vi "Single Step Mode Status.vi"(0 "VISA resource name":refnum<visa-resource-name>, 11 "error in (no error)":errorcluster) -> (4 "VISA resource name out":refnum<visa-resource-name>, 6 "Single Step Mode Status":bool, 15 "error out":errorcluster)   [LabVIEW 2014, in "eec 6700.lvlib"]
doc: "Gets the single step mode status of the power source instrument.\n\nNote : supported in Program mode only."
uses:
  <instrlib>/eec 6700/eec 6700.lvlib
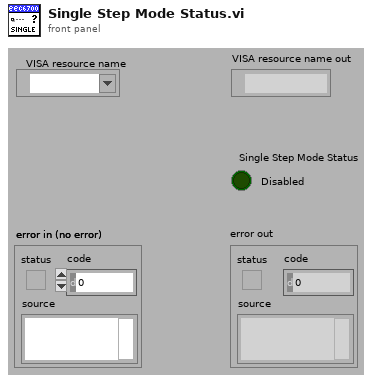
[diagram p1: front panel]
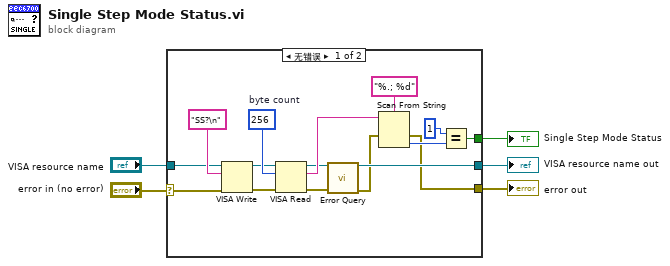
[diagram p0: block diagram]
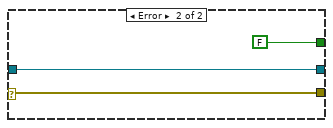
[diagram p2: hidden frame]
diagram:
  n1 = case shown="无错误" "error in (no error)" {
    selector: "error in (no error)" -> [w13 w23]
    tunnel: [w18 FALSE] -> w5
    tunnel: "VISA resource name" -> [w12 w24]
    tunnel: [w6 w23] -> w2
    tunnel: [w10 w24] -> w1
    frame No Error {
      w17 = u32 256  # byte count
      n2 = VISA Write(VISA resource name=w12, write buffer="SS?\n" ("Command to Send (empty)"), error in (no error)=w13) -> (VISA resource name out=w16:refnum<visa-resource-name>, error out=w15:errorcluster)  [unwired: 1 out]
      n3 = VISA Read(VISA resource name=w16, byte count=w17, error in (no error)=w15) -> (VISA resource name out=w9:refnum<visa-resource-name>, read buffer=w11:string, error out=w8:errorcluster)  [unwired: 1 out]
      n4 = call <instrlib>:"Error Query.vi"("VISA resource name"=w9, "error in (no error)"=w8) -> ("VISA resource name out"=w10:refnum<visa-resource-name>, "error out"=w7:errorcluster)  [unwired: 10 in, 2 out]
      n5 = Scan From String(format string="%.; %d" ("Format String"), input string=w11, error in=w7) -> (error out=w6:errorcluster, output 1=w20:i32)  [unwired: 2 in, 2 out]
      n6 = Equal?(x=1, y=w20) -> (x = y?=w18:bool)
    }
    frame Error {
    }
  }
  "Single Step Mode Status" <- w5
  "error out" <- w2
  "VISA resource name out" <- w1
